vi "Controle_camara.vi"(8 "Boolean":bool=TRUE, 11 "time (s) to wait camara":u32=30000) -> (3 "camara":bool)   [LabVIEW 2011]
uses:
  <vilib>/Utility/error.llb/DialogType.ctl
  <vilib>/DAQmx/write.llb/DAQmx Write (Digital Bool 1Line 1Point).vi
  <vilib>/DAQmx/create/channels.llb/DAQmx Create Channel (DO-Digital Output).vi
  <vilib>/DAQmx/miscellaneous.llb/DAQmx Fill In Error Info.vi
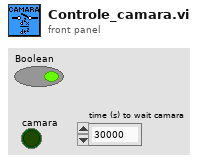
[diagram p1: front panel]
types:
  T1 = typedef "DialogType.ctl" = u16
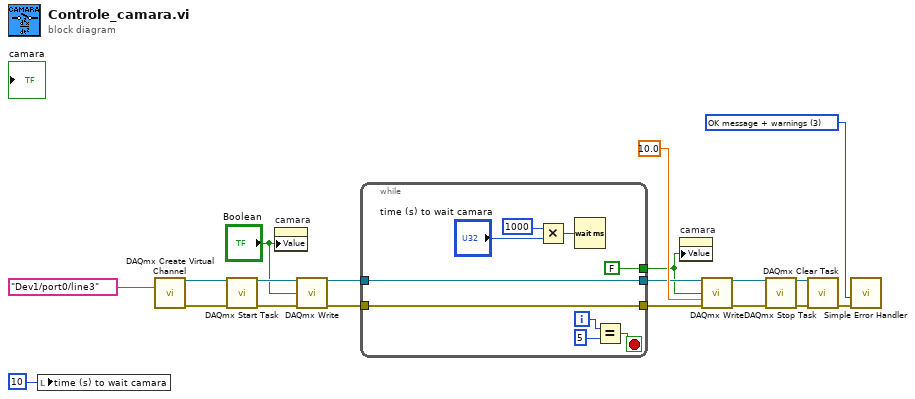
[diagram p0: block diagram]
diagram:
  w16 = T1 3 items=["no dialog", "OK message", "continue or stop message", "OK message + warnings", "continue/stop + warnings"] ("type of dialog (OK msg:1)")
  n1 = local write "time (s) to wait camara"(u32 10 ("time (s) to wait vacuo")) -> ()
  n2 = call-poly <vilib>:"DAQmx Create Virtual Channel.vi"("lines"=tag "Dev1/port0/line3") -> ("task out"=w18:refnum<k21>, "error out"=w17:errorcluster)  [unwired: 13 in]
  n3 = call <vilib>:"DAQmx Start Task.vi"("task/channels in"=w18, "error in"=w17) -> ("task out"=w15:refnum<k21>, "error out"=w14:errorcluster)  [unwired: 12 in]
  n4 = property on="camara" class="Bool (strict)"("Value"="Boolean") -> ()  [unwired: 2 in, 2 out]
  n5 = call-poly <vilib>:"DAQmx Write.vi"("task/channels in"=w15, "data"="Boolean", "error in"=w14) -> ("task out"=w8:refnum<k21>, "error out"=w5:errorcluster)  [unwired: 10 in, 1 out]
  n6 = while {
    tunnel: [FALSE ("Boolean")] -> w2
    tunnel: [w24] -> w7
    tunnel: w8 -> [w24]
    tunnel: [w23] -> w6
    tunnel: w5 -> [w23]
    i -> [w22]
    stop <- w20 stop-if-true
    n7 = Multiply(x=u32 1000, y="time (s) to wait camara") -> (x*y=w26:u32)
    n8 = Wait (ms)(milliseconds to wait=w26) -> ()  [unwired: 1 out]
    n9 = Equal?(x=w22, y=5) -> (x = y?=w20:bool)
  }
  n10 = property on="camara" class="Bool (strict)"("Value"=w2) -> ()  [unwired: 2 in, 2 out]
  n11 = call-poly <vilib>:"DAQmx Write.vi"("task/channels in"=w7, "data"=w2, "timeout"=10.0, "error in"=w6) -> ("task out"=w11:refnum<k21>, "error out"=w10:errorcluster)  [unwired: 9 in, 1 out]
  n12 = call <vilib>:"DAQmx Stop Task.vi"("task/channels in"=w11, "error in"=w10) -> ("task out"=w12:refnum<k21>, "error out"=w13:errorcluster)  [unwired: 12 in]
  n13 = call <vilib>:"DAQmx Clear Task.vi"("task in"=w12, "error in"=w13) -> ("error out"=w19:errorcluster)  [unwired: 13 in]
  n14 = call <vilib>:"Simple Error Handler.vi"("type of dialog (OK msg:1)"=w16, "error in (no error)"=w19) -> ()  [unwired: 3 in, 5 out]
